vi "OAT State Machine Add New Events.vi"(6 "ms timeout (200)":i32=200, 7 "Event Names":string[](array[string]), 8 "queue":T1, 9 "Menu Refnum":refnum<k9>, 10 "New Events":bool[](array[boolean]), 11 "Event Queue In":string[](array[string])) -> (3 "Event Queue Out":string[](array[string]))   [LabVIEW 2017]
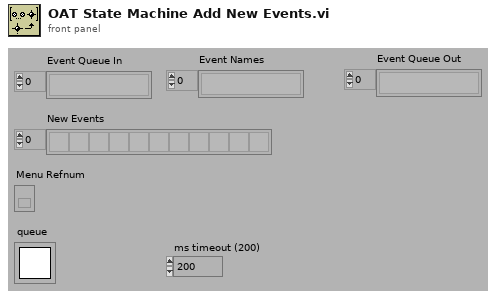
[diagram p1: front panel]
types:
  T1 = typedef "Queue RefNum" = refnum<k1>
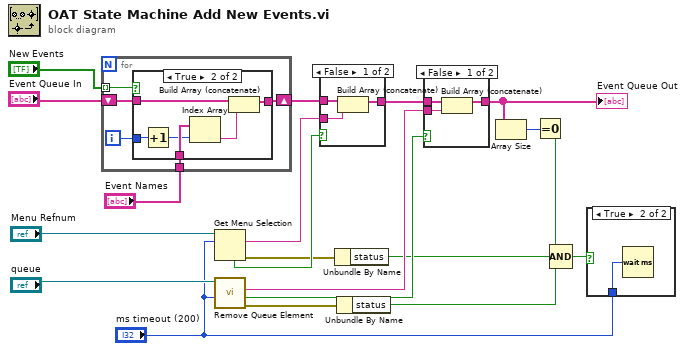
[diagram p0: block diagram]
diagram:
  n1 = for {
    shift-right: [w23] -> w1
    shift-left: "Event Queue In" -> [w24]
    tunnel: "New Events" -> [w22] mode=indexing
    tunnel: "Event Names" -> [w21]
    i -> [w25]
    n2 = case shown="True" w22 {
      tunnel: w25 -> [_ w28]
      tunnel: w24 -> [w26 w32]
      tunnel: [w26 w31] -> w23
      tunnel: w21 -> [_ w29]
      frame False {
      }
      frame True {
        n3 = Increment(x=w28) -> (x+1=w27:i32)
        n4 = Index Array(array=w29, index=w27) -> (element=w30:string)
        n5 = Build Array (concatenate)(w32, w30) -> (w31:string[])
      }
    }
  }
  n6 = Get Menu Selection(0:"Menu Refnum", 1:"ms timeout (200)") -> (4:w15:bool, 6:w13:string, 8:w10:errorcluster)  [unwired: 2 in, 2 out]
  n7 = call <vilib>:"Remove Queue Element.vi"("ms timeout (-1)"="ms timeout (200)", "queue"="queue") -> ("error out"=w9:errorcluster, "timed out"=w11:bool, "queue element"=w14:string)  [unwired: 4 in, 1 out]
  n8 = case shown="False" w15 {
    tunnel: w1 -> [w35 w36]
    tunnel: w13 -> [w34 _]
    tunnel: [w33 w36] -> w12
    frame False {
      n9 = Build Array (concatenate)(w35, w34) -> (w33:string[])
    }
    frame True {
    }
  }
  n10 = Unbundle By Name(w10) -> ("status"=w6:bool)
  n11 = Unbundle By Name(w9) -> ("status"=w5:bool)
  n12 = case shown="False" w11 {
    tunnel: w12 -> [w39 w40]
    tunnel: w14 -> [w38 _]
    tunnel: [w37 w40] -> w2
    frame False {
      n13 = Build Array (concatenate)(w39, w38) -> (w37:string[])
    }
    frame True {
    }
  }
  "Event Queue Out" <- w2
  n14 = Array Size(array=w2) -> (size(s)=w8:i32)
  n15 = Equal To 0?(x=w8) -> (x = 0?=w7:bool)
  n16 = Compound Arithmetic op=AND(w7, w6, w5) -> (w4:bool)
  n17 = case shown="True" w4 {
    tunnel: "ms timeout (200)" -> [_ w41]
    frame False {
    }
    frame True {
      n18 = Wait (ms)(milliseconds to wait=w41) -> ()  [unwired: 1 out]
    }
  }
